vi "禹山浊度_获取温度和测量值.vi"(8 "error in (no error)":errorcluster caption="错误输入（无错误）", 11 "MB session in":refnum<class "MB_Master.lvclass">) -> (0 "error out":errorcluster caption="错误输出", 2 "输出值":cluster{"温度测量值":sgl, "浊度":sgl}, 3 "MB session out":refnum<class "MB_Master.lvclass">)   [LabVIEW 2016, in "斯坦道多参数.lvlib"]
uses:
  <vilib>/Plasmionique/MB Master/MB_Master/MB_Master.lvclass
  <vilib>/Plasmionique/MB Master/MB Master.lvlib
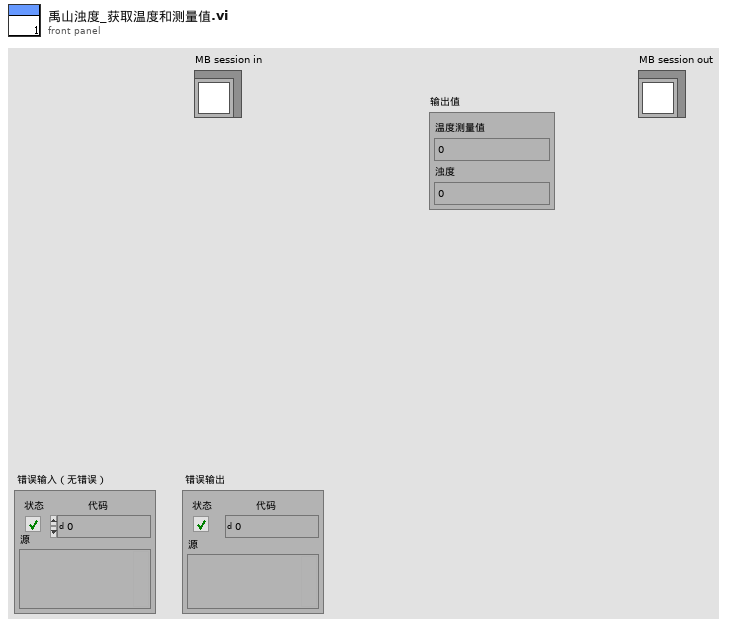
[diagram p1: front panel]
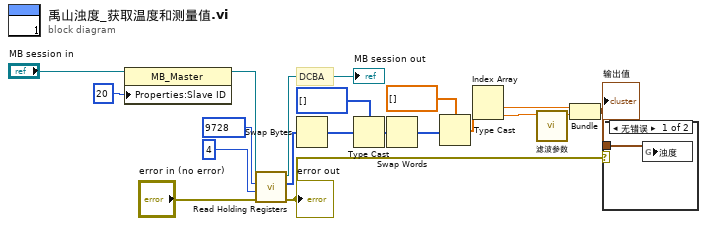
[diagram p0: block diagram]
diagram:
  # "DCBA"
  n1 = property class="MB_Master"(reference="MB session in", "Properties:Slave ID"=u16 20 ("y")) -> (reference out=w11:refnum<class "MB_Master.lvclass">)  [unwired: 1 in, 1 out]
  n2 = call <vilib>:"Read Holding Registers.vi"("error in (no error)"="error in (no error)", "quantity"=u16 4, "starting address"=u16 9728, "MB session in"=w11) -> ("error out"=w6:errorcluster, "Registers"=w9:u16[], "MB session out"=→"MB session out":refnum<class "MB_Master.lvclass">)  [unwired: 5 in]
  "error out" <- w6
  n3 = Swap Bytes(anything=w9) -> (byte swapped=w8:u16[])
  n4 = Type Cast(type=u32[] [] ("数组 2"), x=w8) -> (*(type *) &x=w15:u32[])
  n5 = Swap Words(1:w15) -> (0:w17:u32[])
  n6 = Type Cast(type=sgl[] [] ("数组 2"), x=w17) -> (*(type *) &x=w13:sgl[])
  n7 = Index Array(array=w13) -> (element #1=w7:sgl, element #2=w2:sgl)  [unwired: 2 in]
  n8 = call "滤波参数.vi"("x"=w2) -> ("mode"=w1:dbl)  [unwired: 10 in]
  n9 = Bundle("数值"=w7, "mode"=w1) -> (w5:cluster{"数值":sgl, "mode":dbl})  [unwired: 1 in]
  "输出值" <- w5
  n10 = case shown="无错误" w6 {
    tunnel: w5 -> [w20 _]
    frame No Error {
      n11 = global write "禹山过程全局变量.vi" "浊度"(w20) -> ()
    }
    frame Error {
    }
  }
